vi "MachRampe_ECD.vi"(6 "T_Mach":dbl[](array[numeric]), 7 "t_Mach":dbl[](array[numeric]), 9 "ZykluszeitMod1":dbl, 10 "gleicherZyklus?":i32, 11 "ZeileMach":i32) -> (2 "T_Mach":dbl, 3 "ZeileMach":i32)   [LabVIEW 2017]
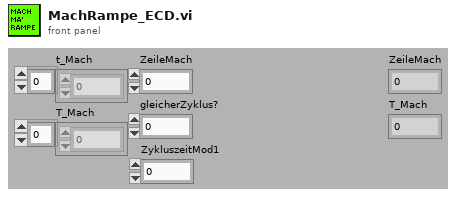
[diagram p1: front panel]
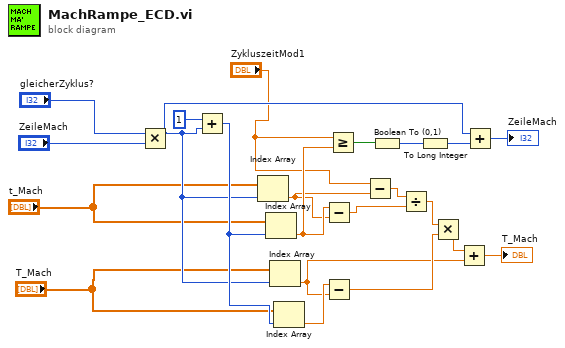
[diagram p0: block diagram]
diagram:
  n1 = Multiply(x="gleicherZyklus?", y="ZeileMach") -> (x*y=w15:i32)
  n2 = Add(x=1 ("y"), y=w15) -> (x+y=w21:i32)
  n3 = Index Array(array="t_Mach", index=w15) -> (element=w14:dbl)
  n4 = Index Array(array="t_Mach", index=w21) -> (element=w19:dbl)
  n5 = Index Array(array="T_Mach", index=w15) -> (element=w8:dbl)
  n6 = Index Array(array="T_Mach", index=w21) -> (element=w20:dbl)
  n7 = Subtract(x=w19, y=w14) -> (x-y=w12:dbl)
  n8 = Subtract(x=w20, y=w8) -> (x-y=w10:dbl)
  n9 = Greater Or Equal?(x="ZykluszeitMod1", y=w19) -> (x >= y?=w18:bool)
  n10 = Subtract(x="ZykluszeitMod1", y=w14) -> (x-y=w13:dbl)
  n11 = Boolean To (0,1)(Boolean=w18) -> (0, 1=w17:i16)
  n12 = Divide(x=w13, y=w12) -> (x/y=w11:dbl)
  n13 = To Long Integer(number=w17) -> (32bit integer=w16:i32)
  n14 = Multiply(x=w11, y=w10) -> (x*y=w9:dbl)
  n15 = Add(x=w9, y=w8) -> (x+y=→"T_Mach":dbl)
  n16 = Add(x=w15, y=w16) -> (x+y=→"ZeileMach":i32)
